vi "Updated Coloured Column.vi"(8 "error in":errorcluster, 11 "MulticolumnListbox in":refnum<vi>) -> (0 "error out":errorcluster, 3 "MulticolumnListbox Out":refnum<vi>)   [LabVIEW 2017, in "DTacq Plot Display Library.lvlib"]
uses:
  DTacq Plot Display Library.lvlib
  <vilib>/Utility/miscctls.llb/LVRowAndColumnTypeDef.ctl
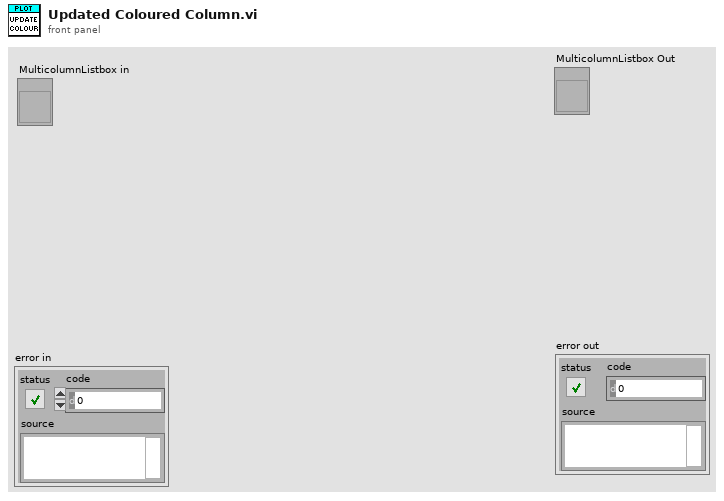
[diagram p1: front panel]
types:
  T1 = typedef "LVRowAndColumnTypeDef.ctl" = cluster{"Row":i32, "Column":i32}
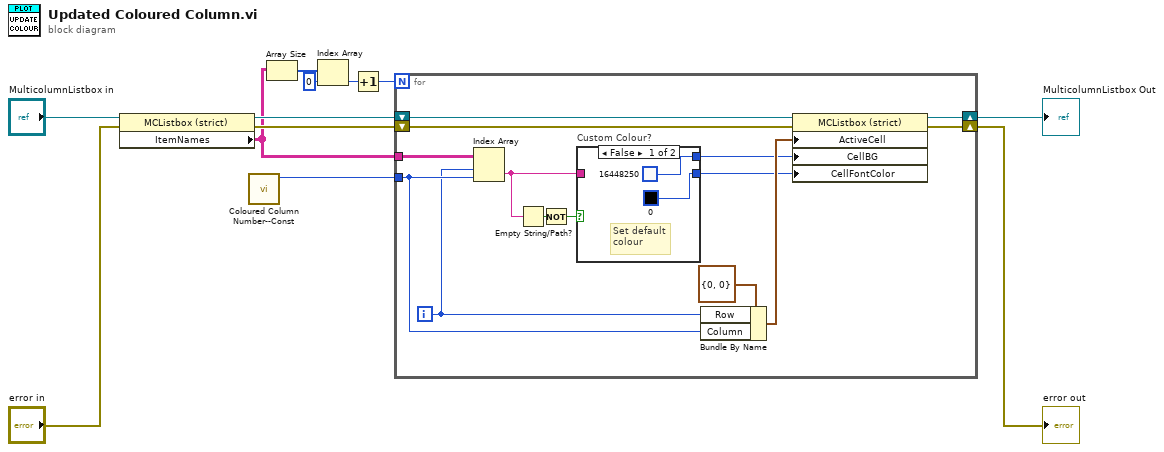
[diagram p0: block diagram]
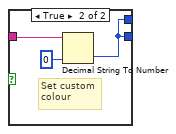
[diagram p2: hidden frame]
diagram:
  n1 = property class="MCListbox (strict)"(reference="MulticolumnListbox in", error in="error in") -> (reference out=w9:refnum<vi>, error out=w8:errorcluster, "ItemNames"=w5:string[][])
  n2 = call "Coloured Column Number--Const.vi"() -> ("Coloured Column"=w10:i32)  [unwired: 11 in]
  n3 = Array Size(array=w5) -> (size(s)=w4:i32[])
  n4 = Index Array(array=w4, index=0) -> (element=w1:i32)
  n5 = Increment(x=w1) -> (x+1=w2:i32)
  n6 = for {
    N: w2 -> [_]
    tunnel: w5 -> [w26]
    tunnel: w10 -> [w24]
    shift-right: [w21] -> w6
    shift-left: w9 -> [w25]
    shift-right: [w20] -> w7
    shift-left: w8 -> [w22]
    i -> [w23]
    n7 = Index Array(array=w26, index (row)=w23, index (col)=w24) -> (element=w19:string)
    n8 = Empty String/Path?(string/path=w19) -> (empty?=w18:bool)
    n9 = Not(x=w18) -> (.not. x?=w15:bool)
    n10 = case "Custom Colour?" shown="False" w15 {
      tunnel: w19 -> [_ w31]
      tunnel: [u32 16448250 w29] -> w14
      tunnel: [u32 0 w29] -> w13
      frame False {
        # "Set default\ncolour"
      }
      frame True {
        # "Set custom\ncolour"
        n11 = Decimal String To Number(string=w31, default (0L)=u32 0 ("Active Cell:Cell Background Color")) -> (number=w29:u32)  [unwired: 1 in, 1 out]
      }
    }
    n12 = Bundle By Name(cluster=T1 {"Row"=0, "Column"=0} ("Active Cell:Active Cell"), "Row"=w23, "Column"=w24) -> (w16:T1)
    n13 = property class="MCListbox (strict)"(reference=w25, error in=w22, "ActiveCell"=w16, "CellBG"=w14, "CellFontColor"=w13) -> (reference out=w21:refnum<vi>, error out=w20:errorcluster)
  }
  "error out" <- w7
  "MulticolumnListbox Out" <- w6
